vi "Open Hardware.vi"(8 "error in (no error)":errorcluster, 11 "Inst.RP100 in":refnum<class "Inst.RP100.lvclass">) -> (0 "error out":errorcluster, 3 "Inst.RP100 out":refnum<class "Inst.RP100.lvclass">)   [LabVIEW 2019, in "Inst.RP100.lvlib" / "Inst.RP100.lvclass"]
uses:
  Inst.RP100.lvclass
  C:/Program Files (x86)/National Instruments/LabVIEW 2019/user.lib/LevyLab/Instrument Framework/Instrument/Instrument.lvclass
  <userlib>/LevyLab/Instrument Framework/Instrument/Instrument.lvclass/Instrument.ctl
  Inst.RP100.lvclass/Inst.RP100.ctl
  <userlib>/LevyLab/Instrument Framework/Instrument Types/Strain/Instrument.Strain.lvclass
  <userlib>/LevyLab/Instrument Framework/Instrument/Instrument.lvclass
  RP100/RP100.lvlib
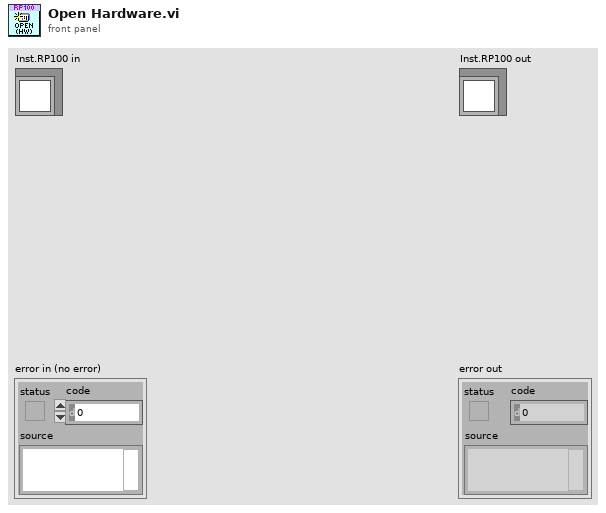
[diagram p1: front panel]
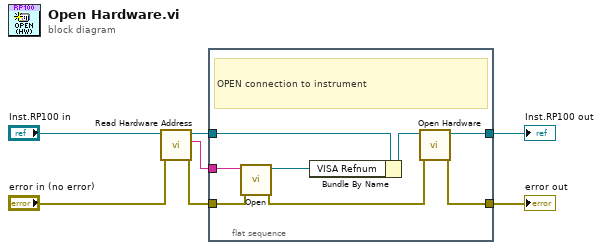
[diagram p0: block diagram]
diagram:
  n1 = call <userlib>:"Read Hardware Address.vi"("error in (no error)"="error in (no error)", "Instrument in"="Inst.RP100 in") -> ("error out"=w5:errorcluster, "Address"=w3:string, "Instrument out"=w2:refnum<class "Inst.RP100.lvclass">)  [unwired: 7 in]
  n2 = flat-sequence {
    tunnel: w2 -> [w15]
    tunnel: [w13] -> w6
    tunnel: w5 -> [w10]
    tunnel: [w12] -> w4
    tunnel: w3 -> [w11]
    frame #0 {
      # "OPEN connection to instrument"
      n3 = call "Open.vi"("error in (no error)"=w10, "VISA resource name"=w11) -> ("error out"=w8:errorcluster, "VISA Refnum out"=w9:refnum<visa-resource-name>)  [unwired: 8 in]
      n4 = Bundle By Name(cluster=w15, "VISA Refnum"=w9) -> (w14:refnum<class "Inst.RP100.lvclass">)
      n5 = call-parent "Open Hardware.vi"("error in (no error)"=w8, "Instrument in"=w14) -> ("error out"=w12:errorcluster, "Instrument out"=w13:refnum<class "Inst.RP100.lvclass">)  [unwired: 8 in]
    }
  }
  "error out" <- w4
  "Inst.RP100 out" <- w6
